vi "Motor-Close.vi"(1 "error out":errorcluster, 2 "MG17Motor 3":refnum<k7>) -> ()   [LabVIEW 2021]
doc: "André Romero - 2016\nandretec@ifsc.usp.br\nIFSC - USP"
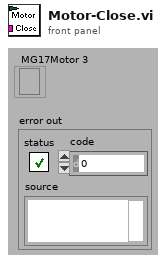
[diagram p1: front panel]
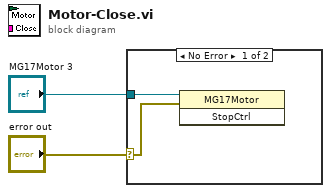
[diagram p0: block diagram]
diagram:
  n1 = case shown="No Error" "error out" {
    selector: "error out" -> [w3 _]
    tunnel: "MG17Motor 3" -> [w4 _]
    frame No Error {
      n2 = invoke class="MG17Motor" method="StopCtrl"(reference=w4, error in=w3) -> ()  [unwired: 1 in, 3 out]
    }
    frame Error {
    }
  }
